vi "Apply Random Factor.vi"(10 "Velocity in":cluster{dbl, dbl}, 11 "AI Manager in":refnum<class "AI Manager.lvclass">) -> (2 "Adjusted Velocity out":cluster{dbl, dbl})   [LabVIEW 2021, in "AI Manager.lvclass"]
doc: "MIT Licence\nCopyright (c) 2024 David Grollier"
uses:
  AI Manager.lvclass
  AI Manager.lvclass/AI Manager.ctl
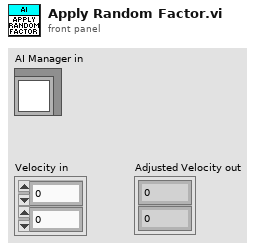
[diagram p1: front panel]
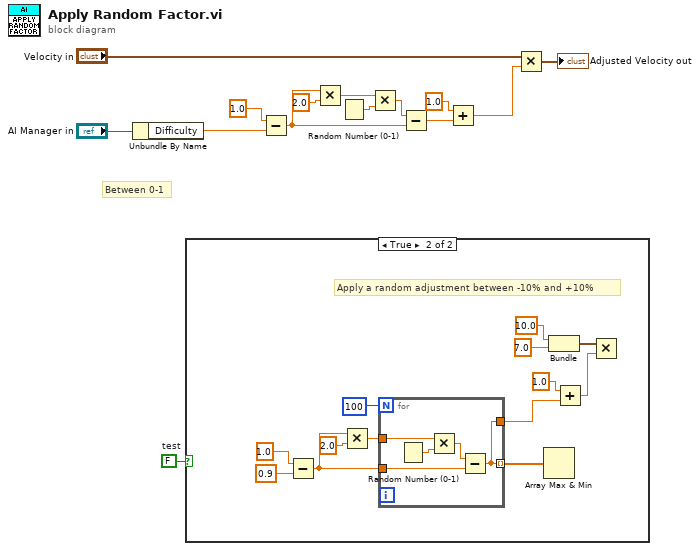
[diagram p0: block diagram]
diagram:
  w4 = FALSE  # test
  # "Between 0-1"
  n1 = Unbundle By Name("AI Manager in") -> ("Difficulty"=w5:dbl)
  n2 = case shown="True" w4 {
    frame False {
    }
    frame True {
      # "Apply a random adjustment between -10% and +10%"
      n3 = Subtract(x=1.0, y=0.9) -> (x-y=w27:dbl)
      n4 = Multiply(x=w27, y=2.0) -> (x*y=w26:dbl)
      n5 = for {
        N: 100 -> [_]
        tunnel: w26 -> [w32]
        tunnel: [w28] -> w22
        tunnel: [w28] -> w16 mode=indexing
        tunnel: w27 -> [w30]
        n6 = Random Number (0-1)() -> (number: 0 to 1=w31:dbl)
        n7 = Multiply(x=w32, y=w31) -> (x*y=w29:dbl)
        n8 = Subtract(x=w29, y=w30) -> (x-y=w28:dbl)
      }
      n9 = Array Max & Min(array=w16) -> ()  [unwired: 4 out]
      n10 = Bundle(10.0, 7.0) -> (w19:cluster{dbl, dbl})  [unwired: 1 in]
      n11 = Add(x=1.0, y=w22) -> (x+y=w23:dbl)
      n12 = Multiply(x=w19, y=w23) -> ()  [unwired: 1 out]
    }
  }
  n13 = Subtract(x=1.0, y=w5) -> (x-y=w7:dbl)
  n14 = Multiply(x=w7, y=2.0) -> (x*y=w8:dbl)
  n15 = Random Number (0-1)() -> (number: 0 to 1=w3:dbl)
  n16 = Multiply(x=w8, y=w3) -> (x*y=w2:dbl)
  n17 = Subtract(x=w2, y=w7) -> (x-y=w10:dbl)
  n18 = Add(x=1.0, y=w10) -> (x+y=w12:dbl)
  n19 = Multiply(x="Velocity in", y=w12) -> (x*y=→"Adjusted Velocity out":cluster{dbl, dbl})
